vi "measurementSetupPanel.vi"() -> ()   [LabVIEW 2013]
uses:
  Controls/instruType.ctl
  Controls/chanType.ctl
  Globals/measurementGlobal.vi
panel:
  in  "Pressure Scanner Clock Chans.":T1(array[cluster])
  in  "Channel Info.":T4(array[cluster]) {"Instru Type" items=["Raw voltage", "Pressure Scanner", "Pressure Transducer", "Pitot-static Tube", "13-Hole Probe"]}
  in  "Input No of Blocks":i32
  in  "Input No of samples":i32
  in  "Input Sampling rate (Hz)":dbl
  in  "NI Device Name":enum16{"USB-6210"}(ring)
  in  "Acquisition Cards":enum16{"NI-USB-6210_Kernel.vi"}(ring)
  in  "Setup":enum16{"Run Programme", "Show Setup"}(ring)
  # "- Add calibration file path\n- Add lab atmospheric information such as (P, T)"
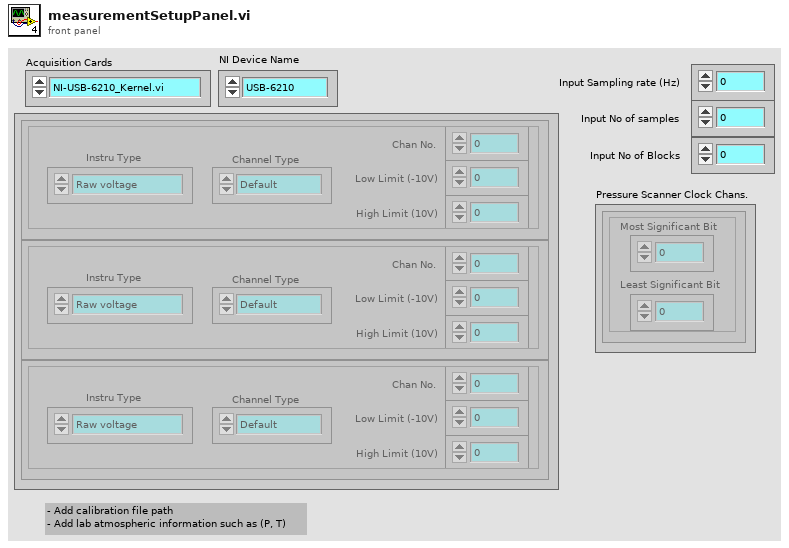
[diagram p1: front panel]
types:
  T1 = cluster{"Least Significant Bit":dbl, "Most Significant Bit":dbl}[]
  T2 = typedef "instruType.ctl" = u16
  T3 = typedef "chanType.ctl" = enum16{"Default", "Clock", "Pressure Scanner"}
  T4 = cluster{"Instru Type":T2, "Channel Type":T3, "Chan No.":i32, "Low Limit (-10V)":dbl, "High Limit (10V)":dbl}[]
  T5 = typedef "chan&Span.ctl" = cluster{"Chan No.":i32, "Low Volt Limit (-10V)":dbl, "High Volt Limit (10V)":dbl, "input terminal configuration":i32}
  T6 = cluster{"Most Significant Bit":dbl, "Least Significant Bit":dbl}[]
  T7 = cluster{"Most Significant Bit":dbl, "Least Significant Bit":dbl}
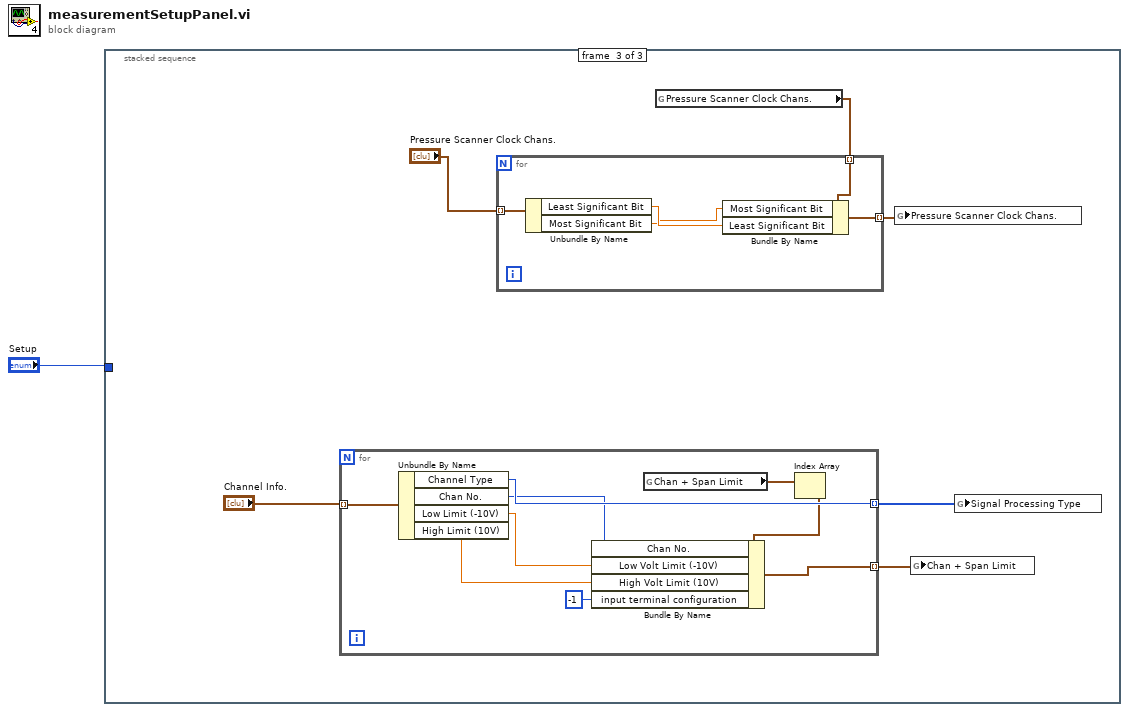
[diagram p0: block diagram]
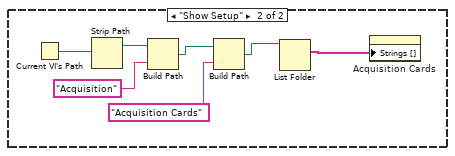
[diagram p3: hidden frame]
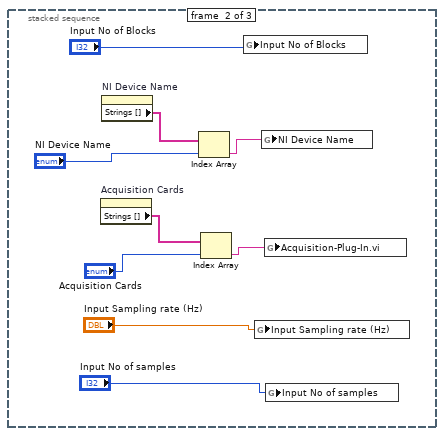
[diagram p4: hidden frame]
diagram:
  n1 = stacked-sequence {
    tunnel: "Setup" -> [w2 _ _]
    frame #0 {
      n2 = case shown="\"Run Programme\", Default" w2 {
        frame "Run Programme", Default {
        }
        frame "Show Setup" {
          n3 = Current VI's Path() -> (path=w9:path)
          n4 = Strip Path(path=w9) -> (stripped path=w8:path)  [unwired: 1 out]
          n5 = Build Path(base path=w8, name or relative path="Acquisition") -> (appended path=w6:path)
          n6 = Build Path(base path=w6, name or relative path="Acquisition Cards") -> (appended path=w4:path)
          n7 = List Folder(path=w4) -> (filenames=w3:string[])  [unwired: 3 in, 3 out]
          n8 = property on="Acquisition Cards" class="Enum (strict)"("Strings []"=w3) -> ()  [unwired: 2 in, 2 out]
        }
      }
    }
    frame #1 {
      n9 = property on="Acquisition Cards" class="Enum (strict)"() -> ("Strings []"=w18:string[])  [unwired: 2 in, 2 out]
      n10 = property on="NI Device Name" class="Enum (strict)"() -> ("Strings []"=w13:string[])  [unwired: 2 in, 2 out]
      n11 = Index Array(array=w13, index="NI Device Name") -> (element=w11:string)
      n12 = Index Array(array=w18, index="Acquisition Cards") -> (element=w16:string)
      n13 = global write "measurementGlobal.vi" "Input No of Blocks"("Input No of Blocks") -> ()
      n14 = global write "measurementGlobal.vi" "Input Sampling rate (Hz)"("Input Sampling rate (Hz)") -> ()
      n15 = global write "measurementGlobal.vi" "NI Device Name"(w11) -> ()
      n16 = global write "measurementGlobal.vi" "Acquisition-Plug-In.vi"(w16) -> ()
      n17 = global write "measurementGlobal.vi" "Input No of samples"("Input No of samples") -> ()
    }
    frame #2 {
      n18 = for {
        tunnel: "Channel Info." -> [w38] mode=indexing
        tunnel: [w37] -> w23 mode=indexing
        tunnel: [w31] -> w19 mode=indexing
        n19 = Unbundle By Name(w38) -> ("Channel Type"=w37:T3, "Chan No."=w36:i32, "Low Limit (-10V)"=w35:dbl, "High Limit (10V)"=w34:dbl)
        n20 = global read "measurementGlobal.vi" "Chan + Span Limit"() -> (w33:T5[])
        n21 = Index Array(array=w33) -> (element=w32:T5)  [unwired: 1 in]
        n22 = Bundle By Name(cluster=w32, "Chan No."=w36, "Low Volt Limit (-10V)"=w35, "High Volt Limit (10V)"=w34, "input terminal configuration"=-1) -> (w31:T5)
      }
      n23 = global read "measurementGlobal.vi" "Pressure Scanner Clock Chans."() -> (w21:T6)
      n24 = for {
        tunnel: "Pressure Scanner Clock Chans." -> [w29] mode=indexing
        tunnel: w21 -> [w28] mode=indexing
        tunnel: [w25] -> w20 mode=indexing
        n25 = Unbundle By Name(w29) -> ("Least Significant Bit"=w27:dbl, "Most Significant Bit"=w26:dbl)
        n26 = Bundle By Name(cluster=w28, "Most Significant Bit"=w26, "Least Significant Bit"=w27) -> (w25:T7)
      }
      n27 = global write "measurementGlobal.vi" "Pressure Scanner Clock Chans."(w20) -> ()
      n28 = global write "measurementGlobal.vi" "Chan + Span Limit"(w19) -> ()
      n29 = global write "measurementGlobal.vi" "Signal Processing Type"(w23) -> ()
    }
  }
